vi "Update Path.vi"(8 "error in (no error)":errorcluster, 10 "Path in":path, 11 "Rename in":refnum<class "ProjectItem.lvclass">) -> (0 "error out":errorcluster, 1 "New Path?":bool, 2 "Path out":path, 3 "Rename out":refnum<class "ProjectItem.lvclass">)   [LabVIEW 2019, in "ProjectItem.lvclass"]
uses:
  ProjectItem.lvclass
  ProjectItem.lvclass/ProjectItem.ctl
  <vilib>/regexp/Match Regular Expression.xnode
panel:
  out "whole match":string
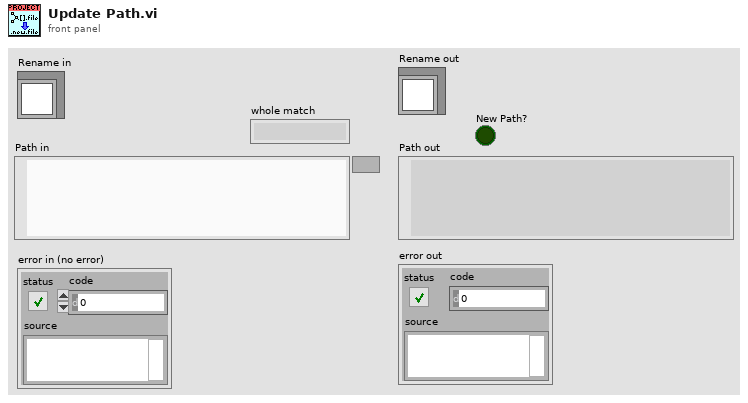
[diagram p1: front panel]
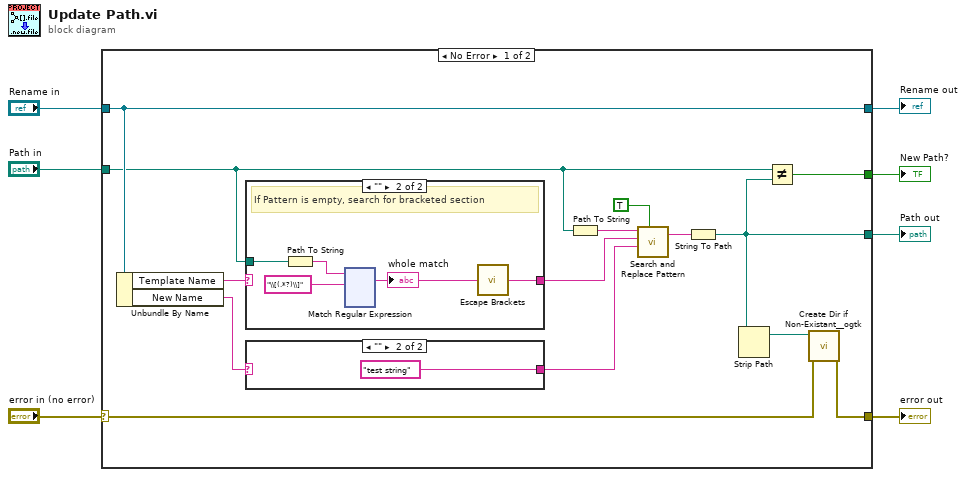
[diagram p0: block diagram]
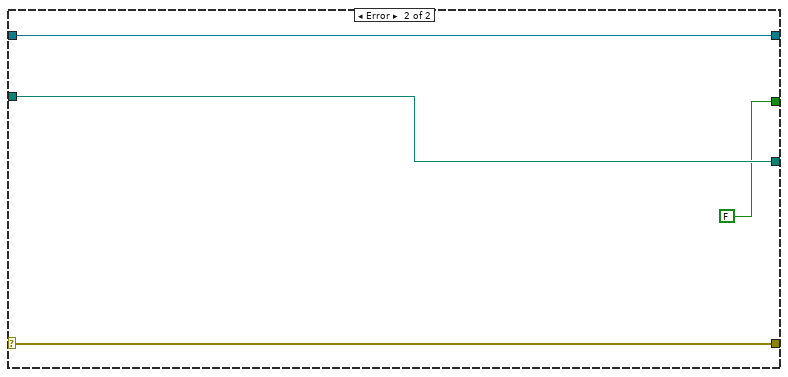
[diagram p4: hidden frame]
diagram:
  n1 = case shown="No Error" "error in (no error)" {
    selector: "error in (no error)" -> [w20 w147]
    tunnel: "Rename in" -> [w21 w146]
    tunnel: [w19 w147] -> w5
    tunnel: [w21 w146] -> w4
    tunnel: [w16 FALSE] -> w2
    tunnel: [w13 w145] -> w3
    tunnel: "Path in" -> [w12 w145]
    frame No Error {
      n2 = Unbundle By Name(w21) -> ("Template Name"=w15:string, "New Name"=w8:string)
      n3 = case shown="\"\"" w15 {
        selector: w15 -> [w24 _]
        tunnel: w12 -> [_ w29]
        tunnel: [w24 w25] -> w14
        frame Default {
        }
        frame "" {
          # "If Pattern is empty, search for bracketed section"
          n4 = Path To String(path=w29) -> (string=w28:string)
          n5 = xnode "Match Regular Expression"("input string"=w28, "regular expression"="\\[(.*?)\\]") -> ("whole match"=w26:string)  [unwired: 4 in, 4 out]
          "whole match" <- w26
          n6 = call "Escape Brackets.vi"("Pattern"=w26) -> ("result string"=w25:string)
        }
      }
      n7 = case shown="\"\"" w8 {
        selector: w8 -> [w22 _]
        tunnel: [w22 "test string"] -> w9
        frame Default {
        }
        frame "" {
        }
      }
      n8 = Path To String(path=w12) -> (string=w11:string)
      n9 = call <vilib>:"Search and Replace Pattern.vi"("string"=w11, "regular expression (\"\")"=w14, "replace string (\"\")"=w9, "replace all? (F)"=TRUE) -> ("result string"=w10:string)  [unwired: 1 in, 1 out]
      n10 = String To Path(string=w10) -> (path=w13:path)
      n11 = Strip Path(path=w13) -> (stripped path=w17:path)  [unwired: 1 out]
      n12 = Not Equal?(x=w12, y=w13) -> (x != y?=w16:bool)
      n13 = call <userlib>:"Create Dir if Non-Existant__ogtk.vi"("error in (no error)"=w20, "Directory Path"=w17) -> ("error out"=w19:errorcluster)  [unwired: 7 in, 2 out]
    }
    frame Error {
    }
  }
  "Rename out" <- w4
  "error out" <- w5
  "Path out" <- w3
  "New Path?" <- w2
